vi "Get Full Decay Fit & Residual Plots (n-Exp Fit) v3.vi"(6 "Fit Options":T12={"Show Fit Residuals"=TRUE, "Fit Model"=enum."1-Exponential", "Residual Type"=enum."Standard", "Max Decay Percentile"=0.0, "Min Decay Percentile"=0.0, "Show Full Decay"=TRUE, "Weights"=enum."Unweighted", "Fitting Method"=enum."Least Square", "Compute Parameter Uncertainties"=TRUE, "Periodic Boundaries"=TRUE, "Model Calculation"=enum."Simulation", "Period"=1.2500000000000001e-08, "Termination Criteria"={"Max Iterations"=1000, "Max Function Calls"=0, "Max Time"=1000.0, "Function Tolerance"=1e-06, "Parameter Tolerance"=1e-06, "Gradient Tolerance"=0.0, "Min Lambda"=1e-06, "Max Lambda"=1e-06, "Initial Tick Count"=0}, "Offset Resolution"=1.2500000000000001e-08, "Use Local IRF"=TRUE, "Fitting Algorithm"=enum."Levenberg-Marquardt", "Show Confidence Interval "=TRUE, "Confidence Level"=95.0} {"Confidence Level" min=0.0 max=100.0; "Offset Resolution" min=0.0; "Period" min=0.0; "Min Decay Percentile" min=0.0 max=1.0; "Max Decay Percentile" min=0.0 max=100.0}, 7 "VI Refnum":refnum<vi>, 8 "Error In":errorcluster, 9 "Fit Output":T1={"best nonlinear fit"=[], "best fit parameters"=[], "R^2"=0.0, "RMSE"=0.0, "error out"={"status"=FALSE, "code"=0, "source"=""}, "Fitting Method"=enum."Least Square", "number of function calls"=0, "number of iterations"=0, "covariance"=[], "Chi 2"=0.0, "DOF"=0, "Fit Convergence Criterion"=enum."Continue", "Fitting Algorithm"=enum."Levenberg-Marquardt", "Weighted Fit"=enum."Unweighted", "Gradient"=0.0, "|Delta Chi 2|"=0.0, "|Delta Chi 2|/Chi 2"=0.0, "Max |Delta a| /|a|"=0.0, "Lambda"=-1.0, "RSS"=0.0, "AIC"=0.0, "BIC"=0.0, "Max number of function calls"=0, "Max number of iterations"=0, "IRF"={"X Array"=[], "Y Array"=[]}, "IRF Normalization Factor"=0.0, "Decay Normalization Factor"=0.0, "Number of offset fits"=0, "Weighted Chi2"=-1.0, "Unweighted Chi2"=-1.0}, 10 "Fit Control Data":T8, 11 "Full Decay":cluster{"t Array":dbl[], "Y Array":dbl[]}) -> (0 "Error Out":errorcluster, 3 "Fit Plots":T11)   [LabVIEW 2021, in "Fits.lvlib"]
uses:
  Fits.lvlib
  Decay Convolution/Decay Model.ctl
  Residual Type.ctl
  Non-linear Fitting Method v2.ctl
  Fit Calculation Method.ctl
  Non-linear Fitting Algorithm.ctl
  Fit Plots.ctl
  Decay Convolution/Fit Control Data v2.ctl
  Graphs/XY Graph/XY Graph Plot Data.ctl
  Decay Fit Parameters In List.ctl
  Non-linear Fit Output v4.ctl
  Nonlinear Fit Method.ctl
  <vilib>/Analysis/Matrix/Datatypes/RealMatrix.ctl
  Convergence Criteria.ctl
  <vilib>/gmath/NumericalOptimization/LM_output select.ctl
  <vilib>/gmath/NI_Gmath.lvlib
  Graphs/XY Graph/XY Graph Add-Ons.lvlib
  <vilib>/Analysis/Matrix/NI_Matrix.lvlib
  Fit Weights Type v2.ctl
  Decay Fit Options v4.ctl
panel:
  out "XY Graph":cluster{"t Array":dbl[], "f(X,a)":dbl[]}[](graph)
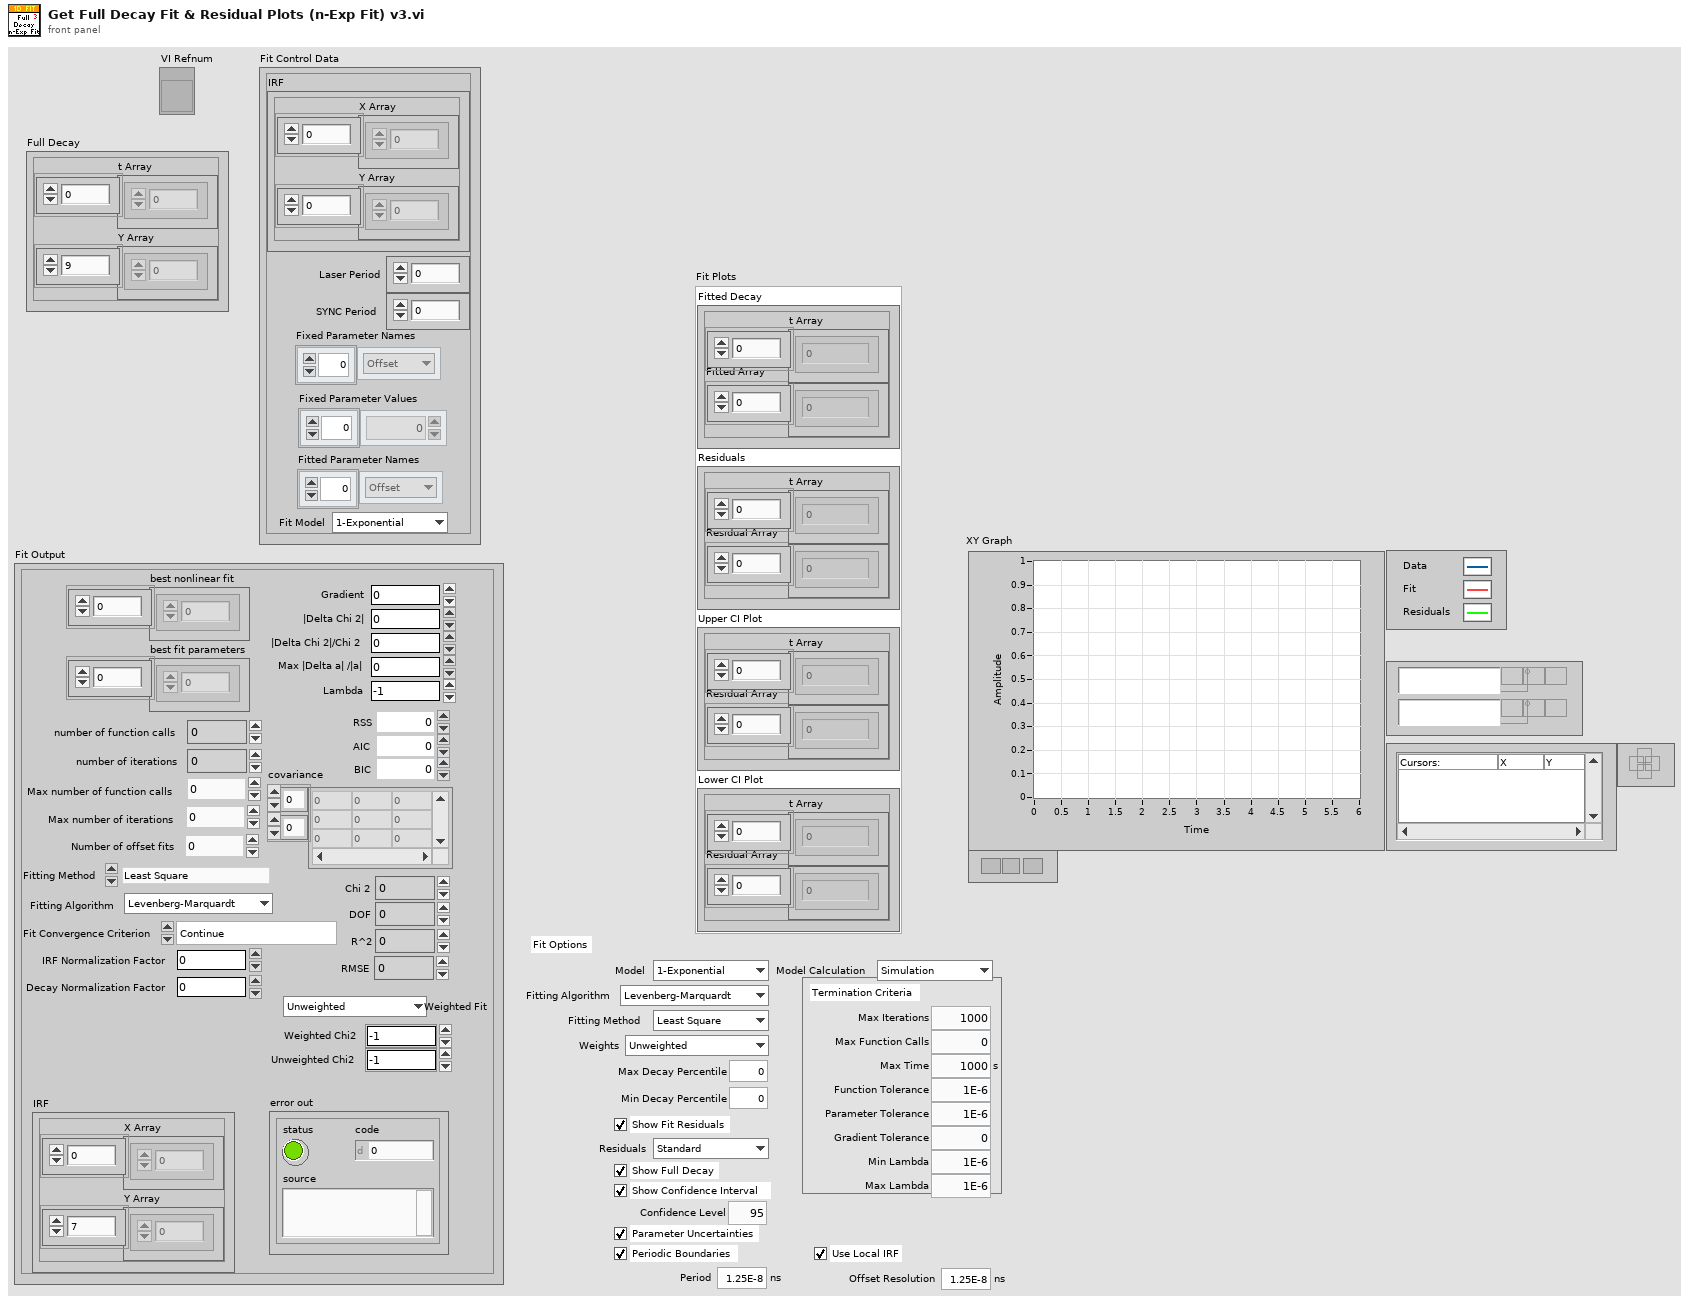
[diagram p1: front panel]
types:
  T1 = typedef "Fits.lvlib/Non-linear Fit Output v4.ctl" = cluster{"best nonlinear fit":dbl[], "best fit parameters":dbl[], "R^2":dbl, "RMSE":dbl, "error out":errorcluster, "Fitting Method":T2, "number of function calls":i32, "number of iterations":i32, "covariance":T3, "Chi 2":dbl, "DOF":i32, "Fit Convergence Criterion":T4, "Fitting Algorithm":T5, "Weighted Fit":T6, "Gradient":dbl, "|Delta Chi 2|":dbl, "|Delta Chi 2|/Chi 2":dbl, "Max |Delta a| /|a|":dbl, "Lambda":dbl, "RSS":dbl, "AIC":dbl, "BIC":dbl, "Max number of function calls":i32, "Max number of iterations":i32, "IRF":T7, "IRF Normalization Factor":dbl, "Decay Normalization Factor":dbl, "Number of offset fits":i32, "Weighted Chi2":dbl, "Unweighted Chi2":dbl}
  T2 = typedef "Fits.lvlib/Nonlinear Fit Method.ctl" = enum16{"Least Square", "Least Absolute Residual", "Bisquare", "MLE"}
  T3 = typedef "NI_Matrix.lvlib/RealMatrix.ctl" = dbl[][]
  T4 = typedef "Fits.lvlib/Convergence Criteria.ctl" = enum16{"Continue", "Tolerances Exceeded", "Max Time Exceeded", "Max Iterations Exceeded", "Max Function Evaluations Exceeded", "Scale Range Exceeded"}
  T5 = typedef "Fits.lvlib/Non-linear Fitting Algorithm.ctl" = enum16{"Levenberg-Marquardt", "Trust-Region Dogleg"}
  T6 = typedef "Fits.lvlib/Fit Weights Type v2.ctl" = enum16{"Unweighted", "1/Variance (Neyman)", "1/Variance (Pearson)", "Best of All"}
  T7 = typedef "XY Graph Add-Ons.lvlib/XY Graph Plot Data.ctl" = cluster{"X Array":dbl[], "Y Array":dbl[]}
  T8 = typedef "Fits.lvlib/Fit Control Data v2.ctl" = cluster{"IRF":T7, "Laser Period":dbl, "SYNC Period":dbl, "Fixed Parameter Names":T9[], "Fixed Parameter Values":dbl[], "Fitted Parameter Names":T9[], "Fit Model":T10}
  T9 = typedef "Fits.lvlib/Decay Fit Parameters In List.ctl" = enum16{"Offset", "Baseline", "A_1", "tau_1", "A_2", "tau_2"}
  T10 = typedef "Fits.lvlib/Decay Model.ctl" = enum16{"1-Exponential", "2-Exponentials"}
  T11 = typedef "Fits.lvlib/Fit Plots.ctl" = cluster{"Fitted Decay":cluster{"t Array":dbl[], "Fitted Array":dbl[]}, "Residuals":cluster{"t Array":dbl[], "Residual Array":dbl[]}, "Upper CI Plot":cluster{"t Array":dbl[], "Residual Array":dbl[]}, "Lower CI Plot":cluster{"t Array":dbl[], "Residual Array":dbl[]}}
  T12 = typedef "Fits.lvlib/Decay Fit Options v4.ctl" = cluster{"Show Fit Residuals":bool, "Fit Model":T10, "Residual Type":T13, "Max Decay Percentile":dbl, "Min Decay Percentile":dbl, "Show Full Decay":bool, "Weights":T6, "Fitting Method":T14, "Compute Parameter Uncertainties":bool, "Periodic Boundaries":bool, "Model Calculation":T15, "Period":dbl[unit], "Termination Criteria":cluster{"Max Iterations":i32, "Max Function Calls":i32, "Max Time":dbl[unit], "Function Tolerance":dbl, "Parameter Tolerance":dbl, "Gradient Tolerance":dbl, "Min Lambda":dbl, "Max Lambda":dbl, "Initial Tick Count":u32}, "Offset Resolution":dbl[unit], "Use Local IRF":bool, "Fitting Algorithm":T5, "Show Confidence Interval ":bool, "Confidence Level":dbl}
  T13 = typedef "Fits.lvlib/Residual Type.ctl" = enum16{"Standard", "Normalized", "Reduced"}
  T14 = typedef "Fits.lvlib/Non-linear Fitting Method v2.ctl" = enum16{"Least Square", "Least Absolute Residual", "Bisquare", "MLE", "-", "Best of All"}
  T15 = typedef "Fits.lvlib/Fit Calculation Method.ctl" = enum16{"Simulation", "Convolution", "Integration"}
  T16 = typedef "NI_Gmath.lvlib/LM_output select.ctl" = cluster{"model function":bool, "gradient":bool}
  T17 = cluster{"VI Refnum":refnum<vi>, "Fit Control Data":T8}
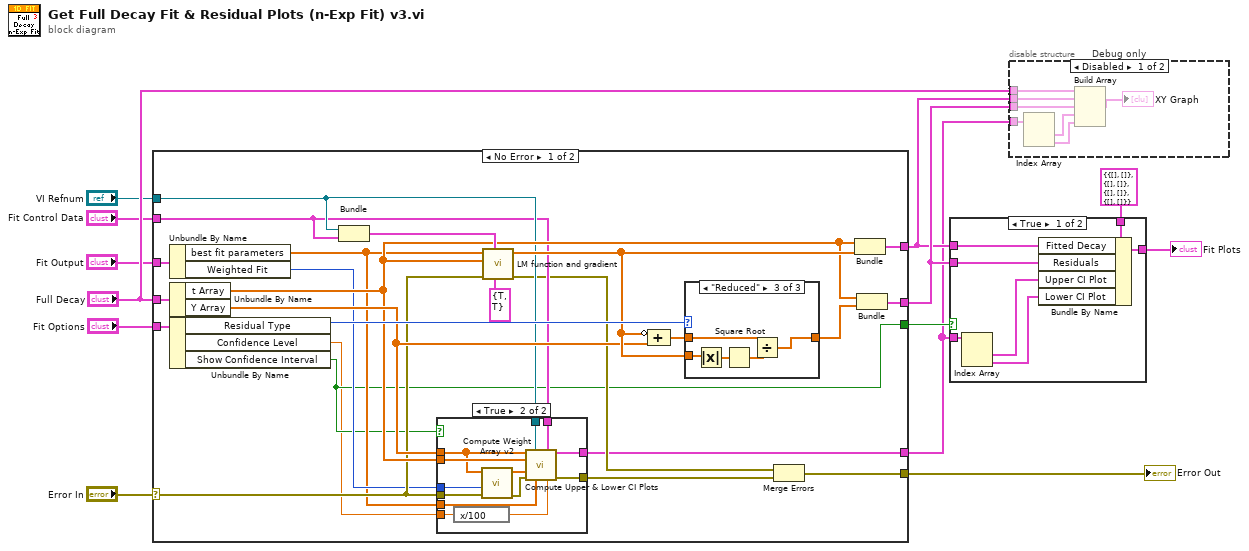
[diagram p0: block diagram]
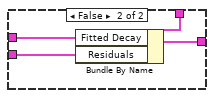
[diagram p2: hidden frame]
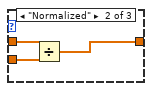
[diagram p6: hidden frame]
diagram:
  n1 = case shown="No Error" "Error In" {
    selector: "Error In" -> [w24 w61]
    tunnel: [w37 _] -> w3
    tunnel: "Fit Options" -> [w36 _]
    tunnel: [w20 w61] -> w12
    tunnel: [w34 _] -> w7
    tunnel: "Full Decay" -> [w33 _]
    tunnel: "Fit Control Data" -> [w22 _]
    tunnel: "VI Refnum" -> [w23 _]
    tunnel: "Fit Output" -> [w28 _]
    tunnel: [w17 _] -> w1
    tunnel: [w15 _] -> w2
    frame No Error {
      n2 = Unbundle By Name(w28) -> ("best fit parameters"=w16:dbl[], "Weighted Fit"=w18:T6)
      n3 = Unbundle By Name(w33) -> ("t Array"=w25:dbl[], "Y Array"=w26:dbl[])
      n4 = Unbundle By Name(w36) -> ("Residual Type"=w31:T13, "Confidence Level"=w14:dbl, "Show Confidence Interval"=w15:bool)
      n5 = Bundle("VI Refnum"=w23, "Fit Control Data"=w22) -> (w30:T17)  [unwired: 1 in]
      n6 = case shown="True" w15 {
        tunnel: w26 -> [_ w44]
        tunnel: w25 -> [_ w51]
        tunnel: w24 -> [w38 w47]
        tunnel: w23 -> [_ w50]
        tunnel: w22 -> [_ w49]
        tunnel: [w38 w48] -> w21
        tunnel: w18 -> [_ w43]
        tunnel: [_ w42] -> w17
        tunnel: w16 -> [_ w41]
        tunnel: w14 -> [_ w40]
        frame False {
        }
        frame True {
          n7 = expression code="x/100"(w40) -> (w39:dbl)
          n8 = call "Compute Weight Array v2.vi"("Error In"=w47, "Weighted Fit"=w43, "Data Array"=w44) -> ("Error Out"=w46:errorcluster, "Weight Array"=w45:dbl[])  [unwired: 7 in]
          n9 = call "Compute Upper & Lower CI Plots.vi"("Y Array"=w44, "VI in"=w50, "Additional LM Data"=w49, "X Array"=w51, "Weight Array"=w45, "error in (no error)"=w46, "best fit parameters"=w41, "confidence level (0.95)"=w39) -> ("CI Plots"=w42:T7[], "error out"=w48:errorcluster)  [unwired: 6 in]
        }
      }
      n10 = call <vilib>:"LM function and gradient.vi"("output control"=T16 {"model function"=TRUE, "gradient"=TRUE}, "model function"=w30, "error in (no error)"=w24, "X"=w25, "a"=w16) -> ("error out"=w19:errorcluster, "f(X)"=w27:dbl[])  [unwired: 3 in, 2 out]
      n11 = Compound Arithmetic op=ADD(invert w27, w26) -> (w32:dbl[])
      n12 = case shown="\"Reduced\"" w31 {
        tunnel: w32 -> [w52 w55 w60]
        tunnel: [w52 w54 w59] -> w35
        tunnel: w27 -> [_ w53 w56]
        frame "Standard", Default {
        }
        frame "Normalized" {
          n13 = Divide(x=w55, y=w53) -> (x/y=w54:dbl[])
        }
        frame "Reduced" {
          n14 = Absolute Value(x=w56) -> (abs(x)=w58:dbl[])
          n15 = Square Root(x=w58) -> (sqrt(x)=w57:dbl[])
          n16 = Divide(x=w60, y=w57) -> (x/y=w59:dbl[])
        }
      }
      n17 = Merge Errors(w19, w21) -> (w20:errorcluster)
      n18 = Bundle("t Array"=w25, "f(X)"=w27) -> (w37:cluster{"t Array":dbl[], "f(X)":dbl[]})  [unwired: 1 in]
      n19 = Bundle("t Array"=w25, w35) -> (w34:cluster{"t Array":dbl[], dbl[]})  [unwired: 1 in]
    }
    frame Error {
    }
  }
  "Error Out" <- w12
  n20 = case shown="True" w2 {
    tunnel: T11 {"Fitted Decay"={"t Array"=[], "Fitted Array"=[]}, "Residuals"={"t Array"=[], "Residual Array"=[]}, "Upper CI Plot"={"t Array"=[], "Residual Array"=[]}, "Lower CI Plot"={"t Array"=[], "Residual Array"=[]}} ("Fit Plots") -> [w68 w72]
    tunnel: [w67 w71] -> w8
    tunnel: w7 -> [w66 w70]
    tunnel: w3 -> [w65 w69]
    tunnel: w1 -> [w64 _]
    frame True {
      n21 = Index Array(array=w64) -> (element #1=w63:T7, element #2=w62:T7)  [unwired: 2 in]
      n22 = Bundle By Name(cluster=w68, "Fitted Decay"=w65, "Residuals"=w66, "Upper CI Plot"=w63, "Lower CI Plot"=w62) -> (w67:T11)
    }
    frame False {
      n23 = Bundle By Name(cluster=w72, "Fitted Decay"=w69, "Residuals"=w70) -> (w71:T11)
    }
  }
  "Fit Plots" <- w8
  n24 = disable-structure "Debug only" shown="Disabled" {
    disable-tunnel: "Full Decay" -> [w79 _]
    disable-tunnel: w3 -> [w77 _]
    disable-tunnel: w7 -> [w76 _]
    disable-tunnel: w1 -> [w75 _]
    frame Disabled {
      n25 = Index Array(array=w75) -> (element #1=w74:T7, element #2=w73:T7)  [unwired: 2 in]
      n26 = Build Array(w79, w77, w76, w74, w73) -> (→"XY Graph":T7[])
    }
    frame Enabled {
    }
  }
